vi "Read Test Case count.vi"(8 "error in (no error)":errorcluster, 11 "Report In":refnum<class "Test Report.lvclass">) -> (0 "error out":errorcluster, 2 "Test Case count":i32, 3 "Report Out":refnum<class "Test Report.lvclass">)   [LabVIEW 2020, in "Test Report.lvclass"]
uses:
  Test Report.lvclass
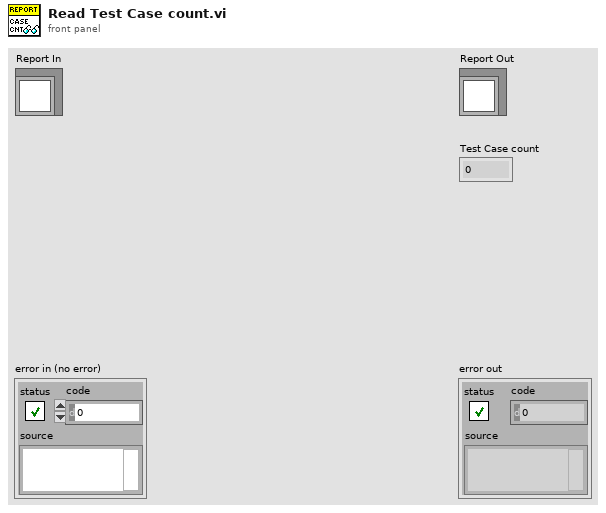
[diagram p1: front panel]
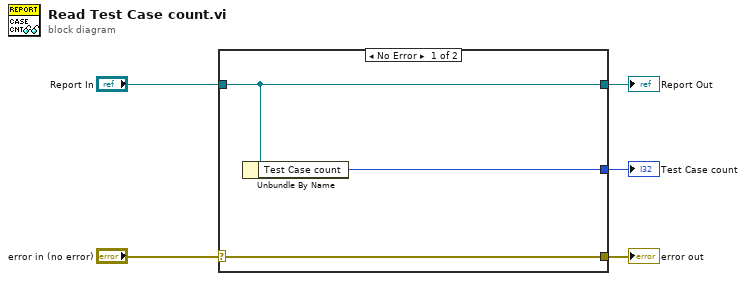
[diagram p0: block diagram]
diagram:
  n1 = case shown="No Error" "error in (no error)" {
    selector: "error in (no error)" -> [w8 w9]
    tunnel: [w8 w9] -> w4
    tunnel: [w7 w10] -> w2
    tunnel: "Report In" -> [w7 w10]
    tunnel: [w6 _] -> w1
    frame No Error {
      n2 = Unbundle By Name(w7) -> ("Test Case count"=w6:i32)
    }
    frame Error {
    }
  }
  "error out" <- w4
  "Report Out" <- w2
  "Test Case count" <- w1
